vi "初始化.vi"() -> (0 "first row":dbl[](array[numeric]) caption="加期限后的日期", 1 "最终选择的真实日期":dbl[](array[numeric]), 2 "密码":string[][](array[string]) caption="所有行")   [LabVIEW 2016]
uses:
  <vilib>/Utility/file.llb/Read Delimited Spreadsheet (DBL).vi
  <vilib>/Utility/file.llb/Read Delimited Spreadsheet (string).vi
  <vilib>/Utility/file.llb/Write Delimited Spreadsheet (DBL).vi
panel:
  out "添加的路径":path
  out "x >= y?":bool
  out "元素 2":dbl
  out "元素":dbl
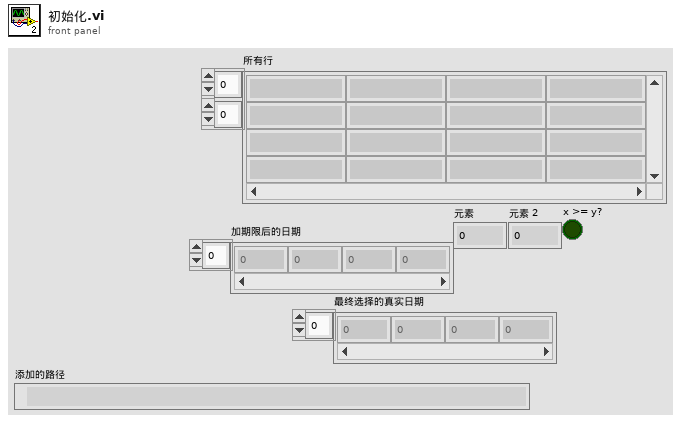
[diagram p1: front panel]
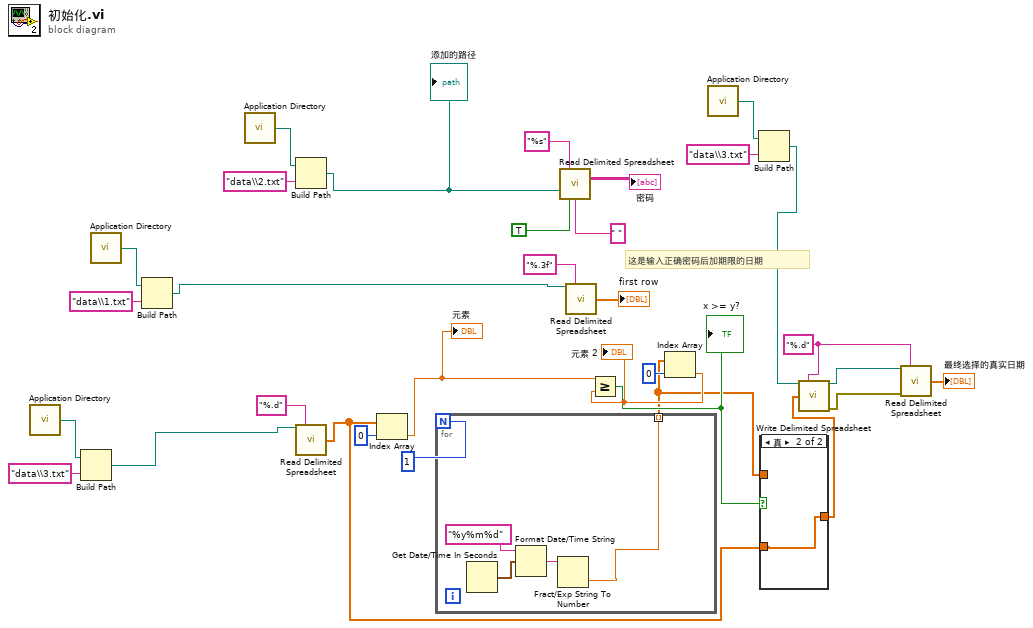
[diagram p0: block diagram]
diagram:
  w22 = "%.d" ("format (%.3f)")
  # "这是输入正确密码后加期限的日期"
  n1 = call <vilib>:"Application Directory.vi"() -> ("Application Directory"=w12:path)
  n2 = Build Path(base path=w12, name or relative path="data\\3.txt" ("名称或相对路径")) -> (appended path=w10:path)
  n3 = call <vilib>:"Application Directory.vi"() -> ("Application Directory"=w5:path)
  n4 = Build Path(base path=w5, name or relative path="data\\1.txt" ("名称或相对路径")) -> (appended path=w4:path)
  n5 = call <vilib>:"Application Directory.vi"() -> ("Application Directory"=w8:path)
  n6 = Build Path(base path=w8, name or relative path="data\\2.txt" ("名称或相对路径")) -> (appended path=w7:path)
  "添加的路径" <- w7
  n7 = call-poly <vilib>:"Read Delimited Spreadsheet.vi"("file path (dialog if empty)"=w10, "format (%.3f)"="%.d") -> ("first row"=w14:dbl[])  [unwired: 8 in, 5 out]
  n8 = Index Array(array=w14, index=0 ("索引")) -> (element=w18:dbl)
  "元素" <- w18
  n9 = for {
    N: 1 -> [_]
    tunnel: [w33] -> w15 mode=indexing
    n10 = Get Date/Time In Seconds() -> (seconds since 1Jan1904=w35:timestamp)
    n11 = Format Date/Time String(time format string (%c)="%y%m%d" ("时间格式字符串(%c)"), seconds (now)=w35) -> (date/time string=w36:string)  [unwired: 1 in]
    n12 = Fract/Exp String To Number(string=w36) -> (number=w33:dbl)  [unwired: 3 in, 1 out]
  }
  n13 = call-poly <vilib>:"Read Delimited Spreadsheet.vi"("file path (dialog if empty)"=w7, "format (%s)"="%s", "transpose? (F)"=TRUE, "delimiter (\\t)"=" " ("delimiter (\\t)")) -> ("all rows"=→"密码":string[][])  [unwired: 6 in, 5 out]
  n14 = call-poly <vilib>:"Read Delimited Spreadsheet.vi"("file path (dialog if empty)"=w4, "format (%.3f)"="%.3f") -> ("first row"=→"first row":dbl[])  [unwired: 8 in, 5 out]
  n15 = Index Array(array=w15, index=0 ("索引")) -> (element=w17:dbl)
  "元素 2" <- w17
  n16 = Greater Or Equal?(x=w18, y=w17) -> (x >= y?=w16:bool)
  "x >= y?" <- w16
  n17 = call <vilib>:"Application Directory.vi"() -> ("Application Directory"=w2:path)
  n18 = Build Path(base path=w2, name or relative path="data\\3.txt" ("名称或相对路径")) -> (appended path=w1:path)
  n19 = case shown="真" w16 {
    tunnel: w15 -> [w37 _]
    tunnel: w14 -> [_ w38]
    tunnel: [w37 w38] -> w13
    frame False {
    }
    frame True {
    }
  }
  n20 = call-poly <vilib>:"Write Delimited Spreadsheet.vi"("file path (dialog if empty)"=w1, "format (%.3f)"=w22, "1D data"=w13) -> ("new file path (Not A Path if cancelled)"=w25:path, "error out"=w24:errorcluster)  [unwired: 11 in]
  n21 = call-poly <vilib>:"Read Delimited Spreadsheet.vi"("file path (dialog if empty)"=w25, "format (%.3f)"=w22, "error in (no error)"=w24) -> ("first row"=→"最终选择的真实日期":dbl[])  [unwired: 7 in, 5 out]
